vi "Create REGISTER msg.vi"(8 "error in (no error)":errorcluster, 10 "REGISTER request data":T1, 11 "Request  ID":u64) -> (0 "error out":errorcluster, 3 "String":string)   [LabVIEW 2020, in "wamplv.lvlib" / "WAMP Client.lvclass"]
uses:
  WAMP Client.lvclass
  TypeDef/REGISTER Request Data.ctl
  TypeDef/Success or error.ctl
  API/TypeDefs/Combined error.ctl
  API/TypeDefs/WAMP error.ctl
  Private/TypeDefs/WAMP Message Codes.ctl
  WAMP Client.lvclass/WAMP Client.ctl
  wamplv.lvlib
  Private/Utils/Utils.lvclass
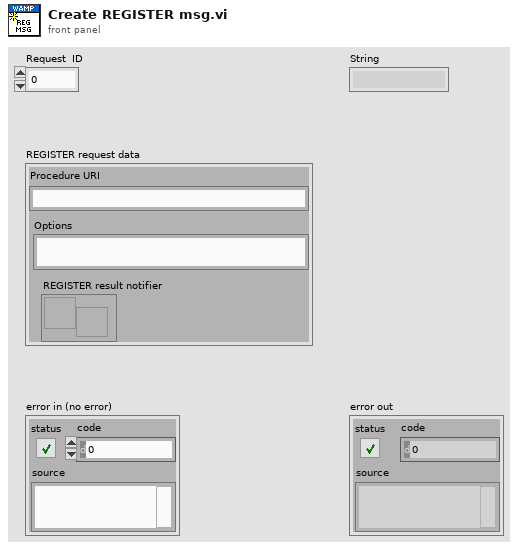
[diagram p1: front panel]
types:
  T1 = typedef "wamplv.lvlib/WAMP Client.lvclass/REGISTER Request Data.ctl" = cluster{"Procedure URI":string, "Options":string, "REGISTER result notifier":refnum<notifier>}
  T2 = typedef "wamplv.lvlib/WAMP Message Codes.ctl" = u16
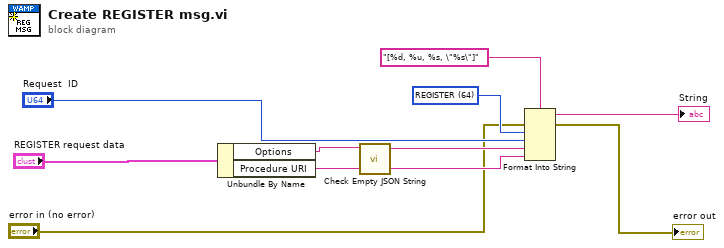
[diagram p0: block diagram]
diagram:
  w5 = T2 64 items=["HELLO"=1, "WELCOME"=2, "ABORT"=3, "GOODBYE"=6, "ERROR"=8, "PUBLISH"=16, "PUBLISHED"=17, "SUBSCRIBE"=32, "SUBSCRIBED"=33, "UNSUBSCRIBE"=34, "UNSUBSCRIBED"=35, "EVENT"=36, "CALL"=48, "RESULT"=59, "REGISTER"=64, "REGISTERED"=65, "UNREGISTER"=66, "UNREGISTERED"=67, "INVOCATION"=68, "YIELD"=70] ("Message Codes")
  n1 = Unbundle By Name("REGISTER request data") -> ("Options"=w8:string, "Procedure URI"=w6:string)
  n2 = call "Check Empty JSON String.vi"("JSON in"=w8) -> ("JSON out"=w9:string)  [unwired: 10 in]
  n3 = Format Into String(format string="[%d, %u, %s, \"%s\"]" ("element"), error in="error in (no error)", w5, "Request  ID", w9, w6) -> (resulting string=→"String":string, error out=→"error out":errorcluster)  [unwired: 1 in]
